vi "Get DescentPoint.vi"(8 "error in (no error)":errorcluster, 10 "Font refnum":refnum<k24>, 11 "String":string) -> (0 "error out":errorcluster, 3 "DescentPoint":sgl)   [LabVIEW 2013]
doc: "Version 1.0\nDeveloped by Jean-Marc Simard\nCopyright © 2010, Exaprom Inc.\nAll rights reserved.\nLicense: BSD\n\nWith iTextSharp 4.1.6 (http://itextsharp.sourceforge.net)\nunder Mozilla Public License Version 1.1\n(http://www.mozilla.org/MPL/MPL-1.1.html)"
uses:
  C:/Users/MaxCorp/Documents/GitHub/TopView/DLL/itextsharp.dll
  DLL/itextsharp.dll
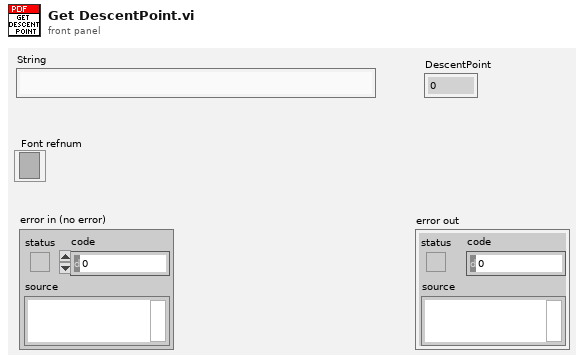
[diagram p1: front panel]
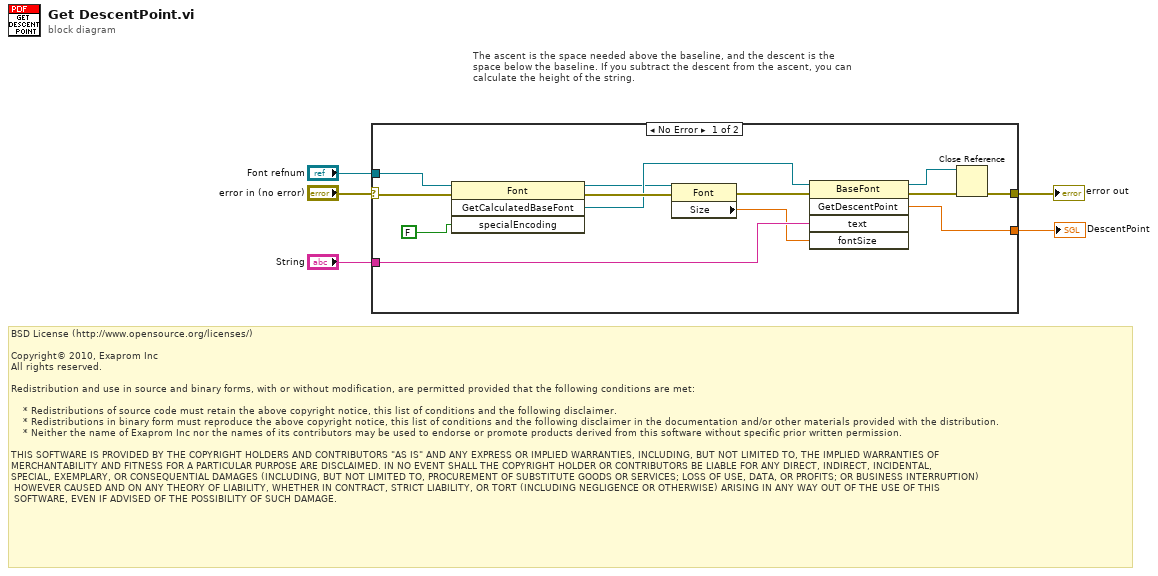
[diagram p0: block diagram]
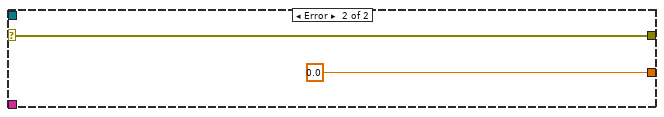
[diagram p2: hidden frame]
diagram:
  # "The ascent is the space needed above the baseline, and the descent is the\nspace below the baseline. If you subtract the descent from the ascent, you can\ncalculate the height of the string."
  # "BSD License (http://www.opensource.org/licenses/)\n\nCopyright© 2010, Exaprom Inc\nAll rights reserved.\n\nRedistribution and use in source and binary forms, with or without modification, are permitted provided that the following conditions are met:\n\n    * Redistributions of source code must retain the above copyright notice, this list of conditions and the following disclaimer.\n    * Redistributions in binary form must reproduce the above copyright notice, this list of conditions and the following disclaimer in the documentation and/or other materials provided with the distribution.\n    * Neither the name of Exaprom Inc nor the names of its contributors may be used to endorse or promote products derived from this software without specific prior written permission.\n\nTHIS SOFTWARE IS PROVIDED BY THE COPYRIGHT HOLDERS AND CONTRIBUTORS \"AS IS\" AND ANY EXPRESS OR IMPLIED WARRANTIES, INCLUDING, BUT NOT LIMITED TO, THE IMPLIED WARRANTIES OF \nMERCHANTABILITY AND FITNESS FOR A PARTICULAR PURPOSE ARE DISCLAIMED. IN NO EVENT SHALL THE COPYRIGHT HOLDER OR CONTRIBUTORS BE LIABLE FOR ANY DIRECT, INDIRECT, INCIDENTAL,\nSPECIAL, EXEMPLARY, OR CONSEQUENTIAL DAMAGES (INCLUDING, BUT NOT LIMITED TO, PROCUREMENT OF SUBSTITUTE GOODS OR SERVICES; LOSS OF USE, DATA, OR PROFITS; OR BUSINESS INTERRUPTION)\n HOWEVER CAUSED AND ON ANY THEORY OF LIABILITY, WHETHER IN CONTRACT, STRICT LIABILITY, OR TORT (INCLUDING NEGLIGENCE OR OTHERWISE) ARISING IN ANY WAY OUT OF THE USE OF THIS\n SOFTWARE, EVEN IF ADVISED OF THE POSSIBILITY OF SUCH DAMAGE."
  n1 = case shown="No Error" "error in (no error)" {
    selector: "error in (no error)" -> [w14 w20]
    tunnel: "String" -> [w17 _]
    tunnel: [w8 w20] -> w4
    tunnel: [w16 sgl 0.0 ("GetDescentPoint")] -> w2
    tunnel: "Font refnum" -> [w15 _]
    frame No Error {
      n2 = invoke class="Font" method="GetCalculatedBaseFont"(reference=w15, error in=w14, "specialEncoding"=FALSE) -> (reference out=w6:refnum<k24>, error out=w13:errorcluster, "GetCalculatedBaseFont"=w11:refnum<k24>)  [unwired: 1 in, 1 out]
      n3 = property class="Font"(reference=w6, error in=w13) -> (error out=w10:errorcluster, "Size"=w12:sgl)  [unwired: 1 out]
      n4 = invoke class="BaseFont" method="GetDescentPoint"(reference=w11, error in=w10, "text"=w17, "fontSize"=w12) -> (reference out=w7:refnum<k24>, error out=w9:errorcluster, "GetDescentPoint"=w16:sgl)  [unwired: 1 in, 2 out]
      n5 = Close Reference(reference=w7, error in (no error)=w9) -> (error out=w8:errorcluster)
    }
    frame Error {
    }
  }
  "error out" <- w4
  "DescentPoint" <- w2
